vi "pH_meter_(Host).vi"() -> ()   [LabVIEW 2013]
doc: "This VI will will initialize the FPGA VI, read calibration values from FPGA, and then continually read single point values from 4 channels of an analog input module."
uses:
  <vilib>/rvi/interface/common/niFpgaWaitOnOcc.vi
  <vilib>/FPGAPlugInAG/myRIO-1900/niLvFpga_Open_myRIO-1900.vi
  <vilib>/rvi/interface/common/dynamic/niFpgaDynamicAddResources.vi
  <vilib>/Utility/error.llb/Error Cluster From Error Code.vi
  <vilib>/rvi/errors/niLvFpgaAdjustHostInterfaceError.vi
  <vilib>/FPGAPlugInAG/Dynamic/niLvFpga_Run_Dynamic.vi
  <vilib>/FPGAPlugInAG/Dynamic/niLvFpga_Close_Dynamic.vi
  <vilib>/rvi/interface/nirviOpenFPGA/nirviOpenFPGA.xnode
  FPGA Bitfiles/myRIOAquaponics_FPGATarget_pHmeter(FPGA)_3EzzEamSfEU.lvbitx
  pH_meter_(FPGA).vi
  <vilib>/rvi/interface/nirviReadWriteControl/nirviReadWriteControl.xnode
  <vilib>/rvi/interface/nirviMethod/nirviMethod.xnode
  <vilib>/rvi/interface/nirviCloseFPGA/nirviCloseFPGA.xnode
  <vilib>/rvi/interface/Simulation/niFpgaSimulationCallBeginRW.vi
  NiFpgaLv.dll
  <vilib>/FPGAPlugInAG/Dynamic/niLvFpga_ConfigureFifo_Dynamic.vi
  <vilib>/rvi/errors/niLvFpgaMergeErrorWithErrorCode.vi
  <vilib>/FPGAPlugInAG/Dynamic/niLvFpga_StartFifo_Dynamic.vi
  <vilib>/FPGAPlugInAG/Dynamic/niLvFpga_ReadFifo_Dynamic.vi
  <vilib>/FPGAPlugInAG/Dynamic/niLvFpga_StopFifo_Dynamic.vi
panel:
  out "PH measurement 2":dbl
  out "Mean (DC)":dbl
  out "Data 4":dbl[](graph)
  in  "stop":bool
  in  "Loop Rate (Hz)":dbl=10000.0
  # "For instructions, select  Help>>Show Context Help and hover over the icon."
  # "Resource Parameters"
  # "Ch 0"
  # "Ch 1"
  # "Ch 2"
  # "Ch 3"
  # "Timing Parameters"
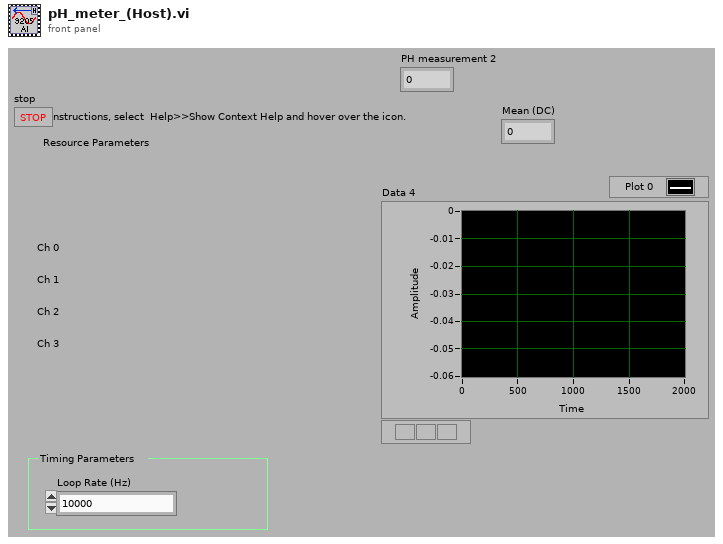
[diagram p1: front panel]
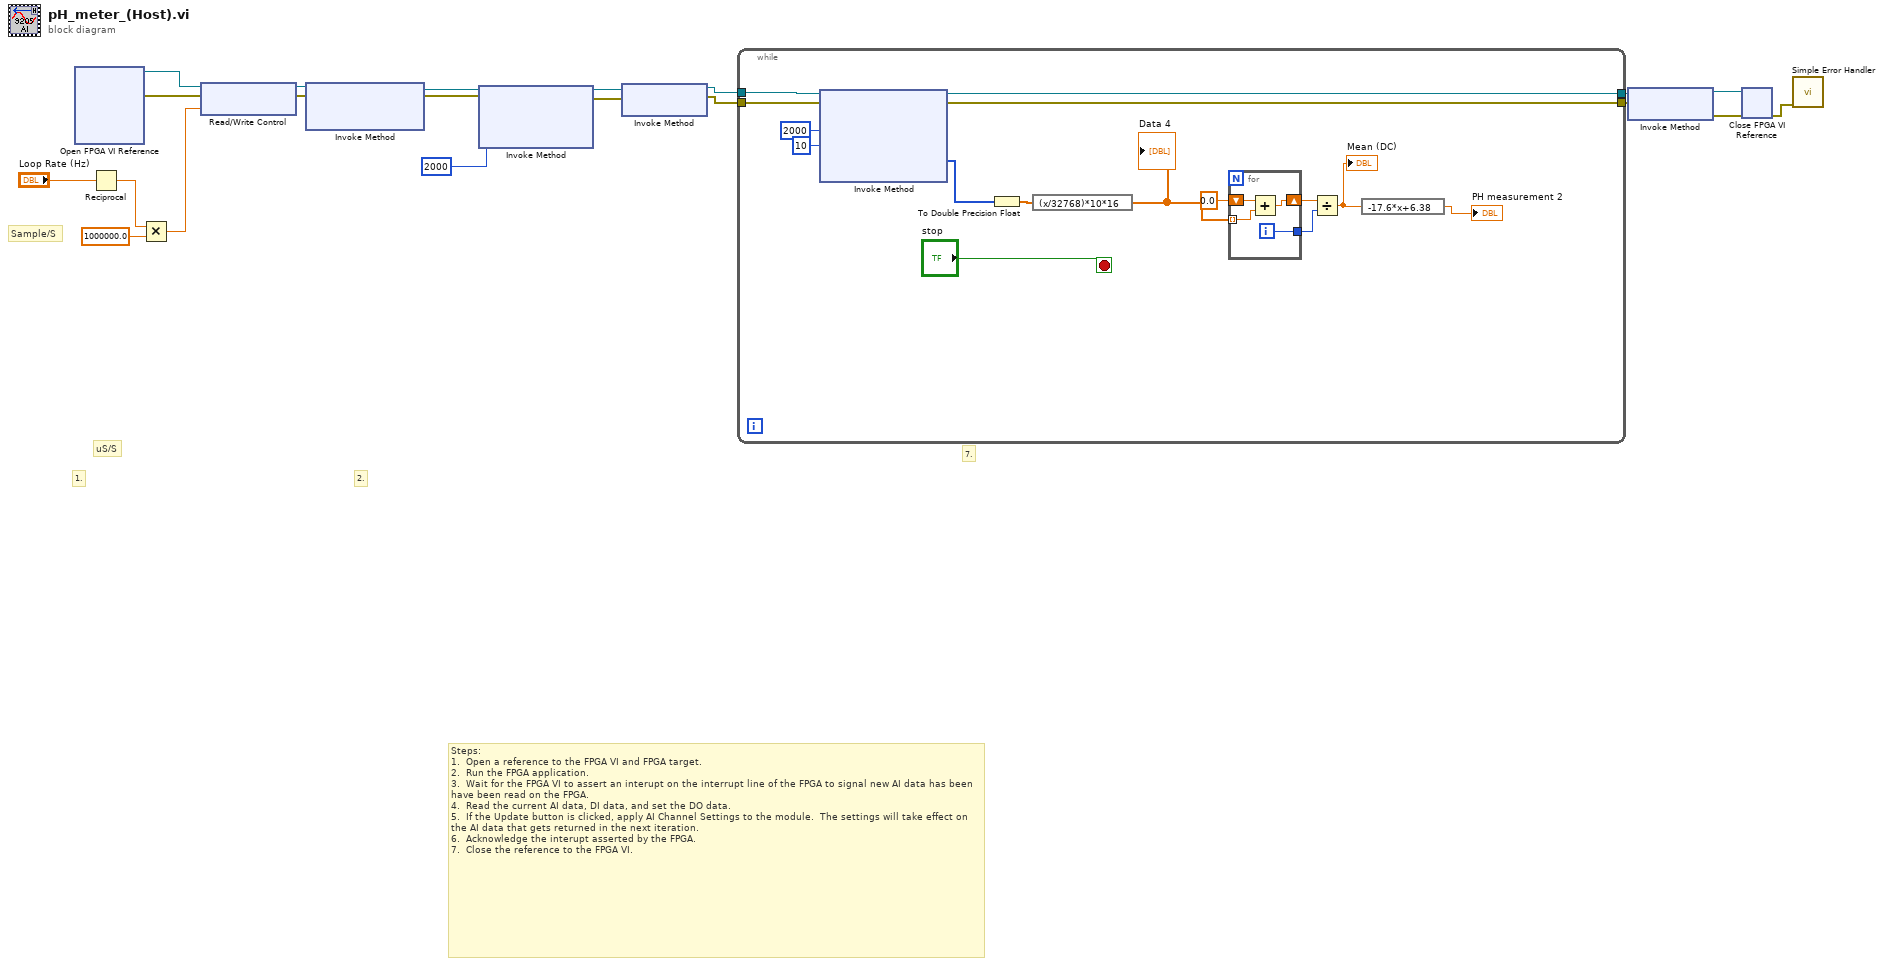
[diagram p0: block diagram]
diagram:
  # "7."
  # "2."
  # "1."
  # "Steps: \n1.  Open a reference to the FPGA VI and FPGA target.\n2.  Run the FPGA application.\n3.  Wait for the FPGA VI to assert an interupt on the interrupt line of the FPGA to signal new AI data has been  have been read on the FPGA.\n4.  Read the current AI data, DI data, and set the DO data.\n5.  If the Update button is clicked, apply AI Channel Settings to the module.  The settings will take effect on the AI data that gets returned in the next iteration.\n6.  Acknowledge the interupt asserted by the FPGA. \n7.  Close the reference to the FPGA VI."
  # "Sample/S"
  # "uS/S"
  n1 = xnode "Open FPGA VI Reference"() -> ("FPGA VI Reference Out"=w13:refnum<k20>, "error out"=w20:errorcluster)  [unwired: 2 in]
  n2 = Reciprocal(x="Loop Rate (Hz)") -> (1/x=w14:dbl)
  n3 = Multiply(x=w14, y=1000000.0) -> (x*y=w12:dbl)
  n4 = xnode "Read/Write Control"("FPGA VI Reference In"=w13, "error in"=w20, "Loop Rate (uS)"=w12) -> ("FPGA VI Reference Out"=w16:refnum<k20>, "error out"=w17:errorcluster)
  n5 = xnode "Invoke Method"("FPGA VI Reference In"=w16, "error in"=w17) -> ("FPGA VI Reference Out"=w11:refnum<k20>, "error out"=w10:errorcluster)  [unwired: 1 in]
  n6 = xnode "Invoke Method"("FPGA VI Reference In"=w11, "error in"=w10, "Requested Depth"=u32 2000) -> ("FPGA VI Reference Out"=w9:refnum<k20>, "error out"=w8:errorcluster)  [unwired: 1 out]
  n7 = xnode "Invoke Method"("FPGA VI Reference In"=w9, "error in"=w8) -> ("FPGA VI Reference Out"=w7:refnum<k20>, "error out"=w6:errorcluster)
  n8 = while {
    tunnel: w7 -> [w35]
    tunnel: w6 -> [w34]
    tunnel: [w33] -> w5
    tunnel: [w32] -> w4
    stop <- "stop" stop-if-true
    n9 = xnode "Invoke Method"("FPGA VI Reference In"=w35, "error in"=w34, "Number of Elements"=u32 2000, "Timeout (ms)"=10) -> ("FPGA VI Reference Out"=w33:refnum<k20>, "error out"=w32:errorcluster, "Data"=w28:i16[])  [unwired: 1 out]
    n10 = To Double Precision Float(number=w28) -> (double precision float=w27:dbl[])
    n11 = expression code="(x/32768)*10*16"(w27) -> (w23:dbl[])
    "Data 4" <- w23
    n12 = for {
      shift-right: [w39] -> w25
      shift-left: 0.0 -> [w37]
      tunnel: [w38] -> w24
      tunnel: w23 -> [w36] mode=indexing
      i -> [w38]
      n13 = Add(x=w37, y=w36) -> (x+y=w39:dbl)
    }
    n14 = Divide(x=w25, y=w24) -> (x/y=w22:dbl)
    "Mean (DC)" <- w22
    n15 = expression code="-17.6*x+6.38"(w22) -> (→"PH measurement 2":dbl)
  }
  n16 = xnode "Invoke Method"("FPGA VI Reference In"=w5, "error in"=w4) -> ("FPGA VI Reference Out"=w3:refnum<k20>, "error out"=w2:errorcluster)
  n17 = xnode "Close FPGA VI Reference"("FPGA VI Reference In"=w3, "error in"=w2) -> ("error out"=w15:errorcluster)
  n18 = call <vilib>:"Simple Error Handler.vi"("error in (no error)"=w15) -> ()  [unwired: 1 in, 8 out]
